vi "__convertUtcTime.vi"(5 "is UTC (F)":bool, 7 "UTC time":timestamp) -> (3 "local time":timestamp)   [LabVIEW 2017]
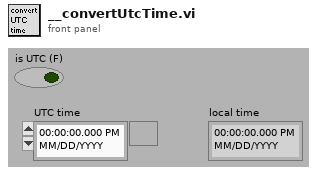
[diagram p1: front panel]
types:
  T1 = typedef "LVDateTimeRec.ctl" = cluster{"fractional second":dbl, "second":i32, "minute":i32, "hour":i32, "day of month":i32, "month":i32, "year":i32, "day of week":i32, "day of year":i32, "DST":i32}
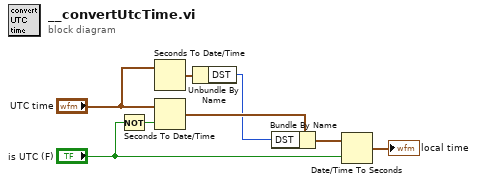
[diagram p0: block diagram]
diagram:
  n1 = Not(x="is UTC (F)") -> (.not. x?=w5:bool)
  n2 = Seconds To Date/Time(time stamp (now)="UTC time") -> (date time rec=w2:T1)  [unwired: 1 in]
  n3 = Seconds To Date/Time(time stamp (now)="UTC time", to UTC (F)=w5) -> (date time rec=w4:T1)
  n4 = Unbundle By Name(w2) -> ("DST"=w1:i32)
  n5 = Bundle By Name(cluster=w4, "DST"=w1) -> (w3:T1)
  n6 = Date/Time To Seconds(1:"is UTC (F)", 2:w3) -> (0:→"local time":timestamp)
